vi "Get VI Name.vi"(11 "Mock VI Call In":refnum<class "Mock VI Call.lvclass">) -> (2 "VI Name":string)   [LabVIEW 2020, in "Mock VI Call.lvclass"]
uses:
  Mock VI Call.lvclass
  Mock VI Call.lvclass/Mock VI Call.ctl
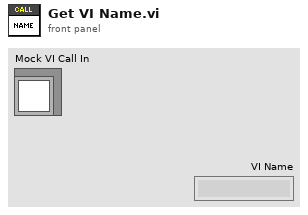
[diagram p1: front panel]
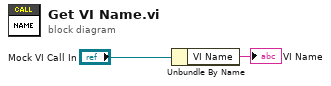
[diagram p0: block diagram]
diagram:
  n1 = Unbundle By Name("Mock VI Call In") -> ("VI Name"=→"VI Name":string)
